vi "ParseAutoScriptText.vi"(11 "output string":string) -> (3 "Array":string[](array[string]))   [LabVIEW 2014]
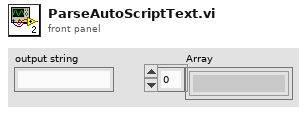
[diagram p1: front panel]
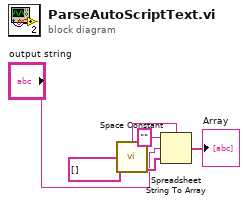
[diagram p0: block diagram]
diagram:
  n1 = call <vilib>:"Space Constant.vi"() -> ("String"=w2:string)
  n2 = Spreadsheet String To Array(delimiter (Tab)=w2, format string="", spreadsheet string="output string", array type (2D Dbl)=string[] []) -> (array=→"Array":string[])
